vi "Convert Item Count to Number String.vi"(11 "Item Count":i32) -> (3 "Number of Items String":string)   [LabVIEW 2020, in "VI Properties Editor.lvlib"]
doc: "Converts <B>Item Count</B> to a string of the form \"# item(s)\" that takes into account whether the word 'item' should be plural or not."
uses:
  VI Properties Editor.lvlib
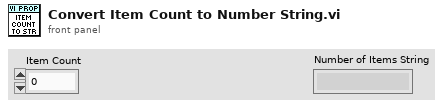
[diagram p1: front panel]
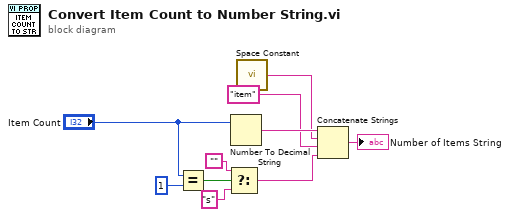
[diagram p0: block diagram]
diagram:
  n1 = Equal?(x="Item Count", y=1) -> (x = y?=w9:bool)
  n2 = Select(t="", s=w9, f="s") -> (s? t:f=w2:string)
  n3 = Number To Decimal String(number="Item Count") -> (decimal integer string=w5:string)  [unwired: 1 in]
  n4 = call <vilib>:"Space Constant.vi"() -> ("String"=w3:string)
  n5 = Concatenate Strings(w5, w3, "item" ("format string"), w2) -> (→"Number of Items String":string)
